vi "CheckIfClassMemberExists.vi"(8 "error in (no error)":errorcluster, 10 "MethodName":string, 11 "LVClassLibrary in":refnum<vi>) -> (0 "error out":errorcluster, 2 "Path":path, 3 "Exists":bool)   [LabVIEW 2020]
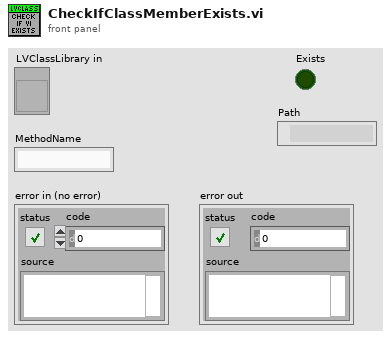
[diagram p1: front panel]
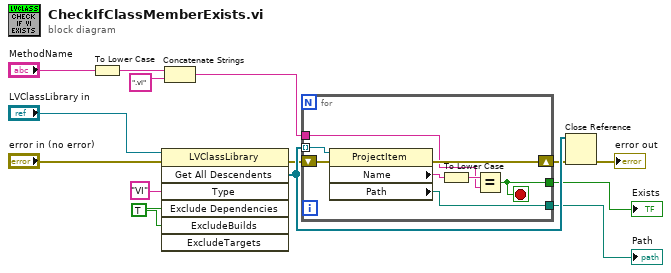
[diagram p0: block diagram]
diagram:
  w14 = TRUE ("ExcludeDependencies")
  n1 = To Lower Case(string="MethodName") -> (all lower case string=w9:string)
  n2 = invoke class="LVClassLibrary" method="Get All Descendents"(reference="LVClassLibrary in", error in="error in (no error)", "Type"="VI", "Exclude Dependencies"=w14, "ExcludeBuilds"=w14) -> (error out=w6:errorcluster, "All Descendents"=w7:refnum<vi>[])  [unwired: 2 in, 5 out]
  n3 = Concatenate Strings(w9, ".vi" ("string")) -> (w3:string)
  n4 = for {
    tunnel: w7 -> [w22] mode=indexing
    tunnel: [w20] -> w1
    shift-right: [w18] -> w5
    shift-left: w6 -> [w19]
    tunnel: w3 -> [w16]
    tunnel: [w15] -> w2
    stop <- w15 stop-if-true
    n5 = property class="ProjectItem"(reference=w22, error in=w19) -> (error out=w18:errorcluster, "Name"=w21:string, "Path"=w20:path)  [unwired: 1 out]
    n6 = To Lower Case(string=w21) -> (all lower case string=w17:string)
    n7 = Equal?(x=w17, y=w16) -> (x = y?=w15:bool)
  }
  "Exists" <- w2
  "Path" <- w1
  n8 = Close Reference(reference=w7, error in (no error)=w5) -> (error out=→"error out":errorcluster)
